vi "KepcoDCPwr Query Output State.vi"(0 "VISA Session":refnum<visa-resource-name>, 1 "Virtual Voltage":dbl format="%.2f", 2 "Virtual Current":dbl format="%.2f", 3 "Virtual Resistance":dbl format="%.2f", 5 "Model In":string, 7 "channel name (\"\")":string="\"\"", 11 "error in (no error)":errorcluster {"code" format="%.0x"}) -> (4 "VISA Session Out":refnum<visa-resource-name>, 6 "Model Out":string, 8 "channel name out (\"\")":string="\"\"" caption="channel name Out (\"\")", 10 "Output state (Constant Voltage)":enum16{"Constatnt Voltage", "Constant Current"}(ring), 15 "error out":errorcluster {"code" format="%.0x"})   [LabVIEW 2020]
doc: "This VI returns whether the power supply is in a particular output state.\n\nA constant voltage condition occurs when the output voltage is equal to the value of the Voltage Level property and the current is less than or equal to the value of the Current Limit property.\n\nA constant current condition occurs when the output current is equal to the value of the Current Limit property."
uses:
  Match Regular Expression.xnode
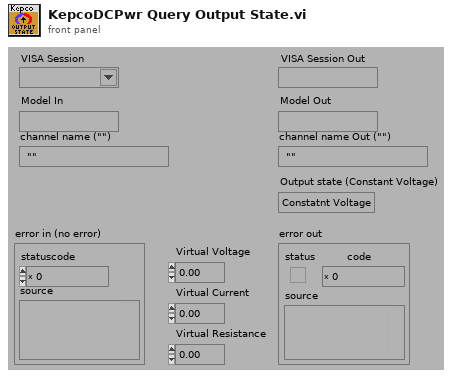
[diagram p1: front panel]
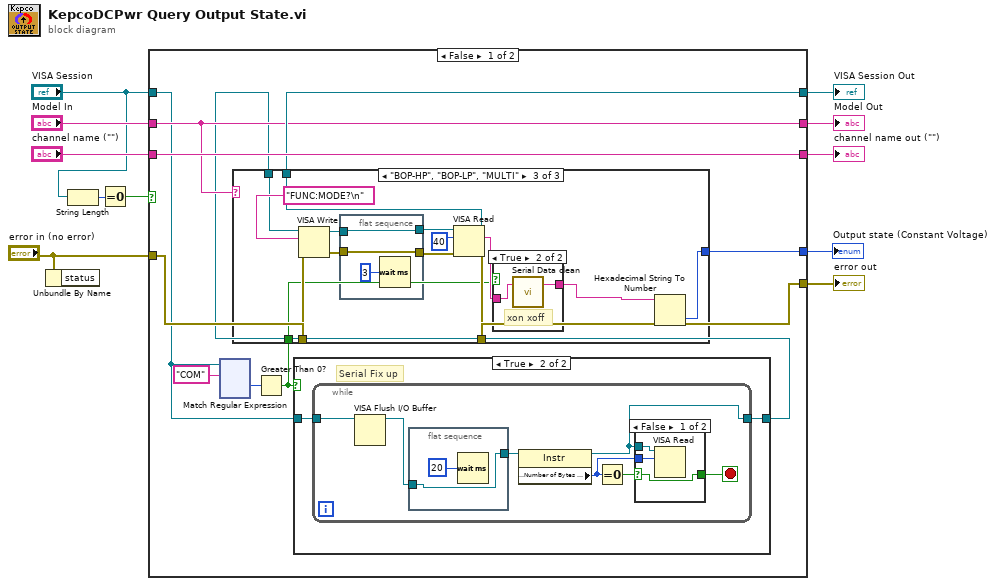
[diagram p0: block diagram]
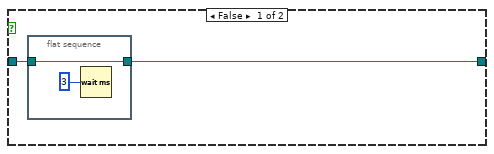
[diagram p2: hidden frame]
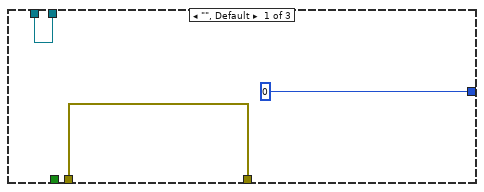
[diagram p4: hidden frame]
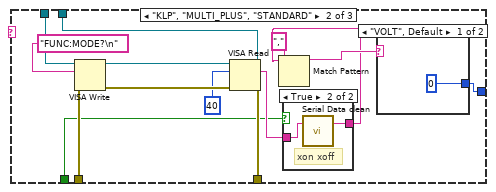
[diagram p5: hidden frame]
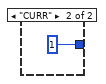
[diagram p7: hidden frame]
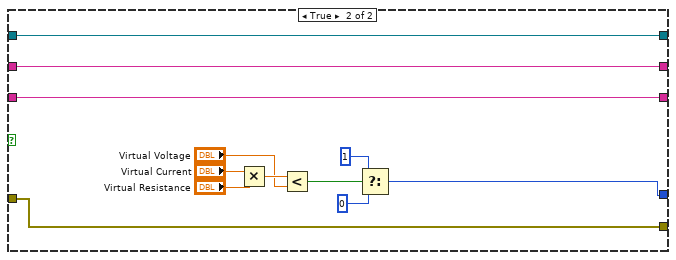
[diagram p9: hidden frame]
diagram:
  n1 = Unbundle By Name("error in (no error)") -> ()  [unwired: 1 out]
  n2 = String Length(string="VISA Session") -> (length=w3:i32)
  n3 = Equal To 0?(x=w3) -> (x = 0?=w1:bool)
  n4 = case shown="False" w1 {
    tunnel: [w18 w206] -> w11
    tunnel: "error in (no error)" -> [w20 w206]
    tunnel: [w21 w205] -> w7
    tunnel: "VISA Session" -> [w14 w205]
    tunnel: [w19 w204] -> w6
    tunnel: "Model In" -> [w19 w204]
    tunnel: [w22 w203] -> w5
    tunnel: "channel name (\"\")" -> [w22 w203]
    tunnel: [w17 w200] -> w4
    frame False {
      n5 = xnode "Match Regular Expression"("input string"=w14, "regular expression"="COM") -> ("offset past match"=w15:i32)  [unwired: 2 in, 6 out]
      n6 = Greater Than 0?(x=w15) -> (x > 0?=w12:bool)
      n7 = case shown="True" w12 {
        tunnel: [w24 w28] -> w13
        tunnel: w14 -> [w23 w27]
        frame False {
          n8 = flat-sequence {
            tunnel: w23 -> [w26]
            tunnel: [w26] -> w24
            frame #0 {
              n9 = Wait (ms)(milliseconds to wait=u32 3 ("byte count (0)")) -> ()  [unwired: 1 out]
            }
          }
        }
        frame True {
          # "Serial Fix up"
          n10 = while {
            tunnel: w27 -> [w31]
            tunnel: [w33] -> w28
            stop <- w34 stop-if-true
            n11 = VISA Flush I/O Buffer(VISA resource name=w31) -> (VISA resource name out=w30:refnum<visa-resource-name>)  [unwired: 2 in, 1 out]
            n12 = flat-sequence {
              tunnel: w30 -> [w36]
              tunnel: [w36] -> w29
              frame #0 {
                n13 = Wait (ms)(milliseconds to wait=u32 20) -> ()  [unwired: 1 out]
              }
            }
            n14 = property class="Instr"(reference=w29) -> (reference out=w33:refnum<visa-resource-name>, "Serial Settings:Number of Bytes at Serial Port"=w32:u32)  [unwired: 1 in, 1 out]
            n15 = Equal To 0?(x=w32) -> (x = 0?=w35:bool)
            n16 = case shown="False" w35 {
              selector: w35 -> [w40 w41]
              tunnel: [w40 w41] -> w34
              tunnel: w33 -> [w39 _]
              tunnel: w32 -> [w38 _]
              frame False {
                n17 = VISA Read(VISA resource name=w39, byte count=w38) -> ()  [unwired: 1 in, 4 out]
              }
              frame True {
              }
            }
          }
        }
      }
      n18 = case shown="\"BOP-HP\", \"BOP-LP\", \"MULTI\"" w19 {
        tunnel: w20 -> [w155 w169 w188]
        tunnel: [w155 w163 w184] -> w18
        tunnel: [w154 w165 w185] -> w21
        tunnel: w13 -> [w154 w167 w186]
        tunnel: [0 w159 w175] -> w17
        tunnel: w12 -> [_ w156 w177]
        frame "", Default {
        }
        frame "KLP", "MULTI_PLUS", "STANDARD" {
          n19 = VISA Write(VISA resource name=w167, write buffer="FUNC:MODE?\n", error in (no error)=w169) -> (VISA resource name out=w164:refnum<visa-resource-name>, error out=w166:errorcluster)  [unwired: 1 out]
          n20 = VISA Read(VISA resource name=w164, byte count=u32 40 ("byte count (0)"), error in (no error)=w166) -> (VISA resource name out=w165:refnum<visa-resource-name>, read buffer=w158:string, error out=w163:errorcluster)  [unwired: 1 out]
          n21 = case shown="True" w156 {
            tunnel: [w170 w171] -> w157
            tunnel: w158 -> [w170 w172]
            frame False {
            }
            frame True {
              # "xon xoff"
              n22 = call "Serial Data clean.vi"("string"=w172) -> ("Stripped of Xon Xoff"=w171:string)  [unwired: 2 in]
            }
          }
          n23 = Match Pattern(string=w157, regular expression=",") -> (before substring=w160:string)  [unwired: 4 out]
          n24 = case shown="\"VOLT\", Default" w160 {
            tunnel: [0 1] -> w159
            frame "VOLT", Default {
            }
            frame "CURR" {
            }
          }
        }
        frame "BOP-HP", "BOP-LP", "MULTI" {
          n25 = VISA Write(VISA resource name=w186, write buffer="FUNC:MODE?\n", error in (no error)=w188) -> (VISA resource name out=w182:refnum<visa-resource-name>, error out=w180:errorcluster)  [unwired: 1 out]
          n26 = flat-sequence {
            tunnel: [w194] -> w181
            tunnel: w182 -> [w194]
            tunnel: [w192] -> w179
            tunnel: w180 -> [w192]
            frame #0 {
              n27 = Wait (ms)(milliseconds to wait=u32 3 ("byte count (0)")) -> ()  [unwired: 1 out]
            }
          }
          n28 = VISA Read(VISA resource name=w181, byte count=u32 40 ("byte count (0)"), error in (no error)=w179) -> (VISA resource name out=w185:refnum<visa-resource-name>, read buffer=w178:string, error out=w184:errorcluster)  [unwired: 1 out]
          n29 = case shown="True" w177 {
            tunnel: [w189 w190] -> w176
            tunnel: w178 -> [w189 w191]
            frame False {
            }
            frame True {
              # "xon xoff"
              n30 = call "Serial Data clean.vi"("string"=w191) -> ("Stripped of Xon Xoff"=w190:string)  [unwired: 2 in]
            }
          }
          n31 = Hexadecimal String To Number(string=w176) -> (number=w175:u32)  [unwired: 2 in, 1 out]
        }
      }
    }
    frame True {
      n32 = Multiply(x="Virtual Current", y="Virtual Resistance") -> (x*y=w197:dbl)
      n33 = Less?(x=w197, y="Virtual Voltage") -> (x < y?=w195:bool)
      n34 = Select(t=1, s=w195, f=0) -> (s? t:f=w200:i32)
    }
  }
  "error out" <- w11
  "channel name out (\"\")" <- w5
  "Model Out" <- w6
  "VISA Session Out" <- w7
  "Output state (Constant Voltage)" <- w4
